vi "VL6180 GetRegister.vi"(7 "VL6180 Resource":T8 {"I2C Slave Address" format="%02x"}, 8 "error in":errorcluster, 10 "VL6180X Constants":T7 items=["IDENTIFICATION_MODEL_ID"=0, "IDENTIFICATION_MODEL_REV_MAJOR"=1, "IDENTIFICATION_MODEL_REV_MINOR"=2, "IDENTIFICATION_MODULE_REV_MAJOR"=3, "IDENTIFICATION_MODULE_REV_MINOR"=4, "IDENTIFICATION_DATE"=6, "IDENTIFICATION_TIME"=8, "SYSTEM_MODE_GPIO0"=16, "SYSTEM_MODE_GPIO1"=17, "SYSTEM_HISTORY_CTRL"=18, "SYSTEM_INTERRUPT_CONFIG_GPIO"=20, "SYSTEM_INTERRUPT_CLEAR"=21, "SYSTEM_FRESH_OUT_OF_RESET"=22, "SYSTEM_GROUPED_PARAMETER_HOLD"=23, "SYSRANGE_START"=24, "SYSRANGE_THRESH_HIGH"=25, "SYSRANGE_THRESH_LOW"=26, "SYSRANGE_INTERMEASUREMENT_PERIOD"=27, "SYSRANGE_MAX_CONVERGENCE_TIME"=28, "SYSRANGE_CROSSTALK_COMPENSATION_RATE"=30, "SYSRANGE_CROSSTALK_VALID_HEIGHT"=33, "SYSRANGE_EARLY_CONVERGENCE_ESTIMATE"=34, "SYSRANGE_PART_TO_PART_RANGE_OFFSET"=36, "SYSRANGE_RANGE_IGNORE_VALID_HEIGHT"=37, "SYSRANGE_RANGE_IGNORE_THRESHOLD"=38, "SYSRANGE_MAX_AMBIENT_LEVEL_MULT"=44, "SYSRANGE_RANGE_CHECK_ENABLES"=45, "SYSRANGE_VHV_RECALIBRATE"=46, "SYSRANGE_VHV_REPEAT_RATE"=49, "SYSALS_START"=56, "SYSALS_THRESH_HIGH"=58, "SYSALS_THRESH_LOW"=60, "SYSALS_INTERMEASUREMENT_PERIOD"=62, "SYSALS_ANALOGUE_GAIN"=63, "SYSALS_INTEGRATION_PERIOD"=64, "RESULT_RANGE_STATUS"=77, "RESULT_ALS_STATUS"=78, "RESULT_INTERRUPT_STATUS_GPIO"=79, "RESULT_ALS_VAL"=80, "RESULT_HISTORY_BUFFER"=82, "RESULT_RANGE_VAL"=98, "RESULT_RANGE_RAW"=100, "RESULT_RANGE_RETURN_RATE"=102, "RESULT_RANGE_REFERENCE_RATE"=104, "RESULT_RANGE_RETURN_SIGNAL_COUNT"=108, "RESULT_RANGE_REFERENCE_SIGNAL_COUNT"=112, "RESULT_RANGE_RETURN_AMB_COUNT"=116, "RESULT_RANGE_REFERENCE_AMB_COUNT"=120, "RESULT_RANGE_RETURN_CONV_TIME"=124, "RESULT_RANGE_REFERENCE_CONV_TIME"=128, "READOUT_AVERAGING_SAMPLE_PERIOD"=266, "FIRMWARE_BOOTUP"=281, "FIRMWARE_RESULT_SCALER"=288, "I2C_SLAVE_DEVICE_ADDRESS"=530, "INTERLEAVED_MODE_ENABLE"=675], 11 "LINX Resource":T1) -> (0 "error out":errorcluster, 2 "Data out":u8 format="%02x", 3 "LINX Resource":T1, 5 "VL6180 Resource":T8 {"I2C Slave Address" format="%02x"})   [LabVIEW 2014]
uses:
  VL6180 Resource.ctl
  VL6180X DEFS.ctl
  <vilib>/MakerHub/LINX/Private/Type Defs/LINX Ref.ctl
  <vilib>/MakerHub/LINX/Private/Type Defs/Platform.ctl
  <vilib>/MakerHub/LINX/Private/Type Defs/Interface.ctl
  <vilib>/MakerHub/LINX/Private/Device/Type Defs/LINX Device Config.ctl
  <vilib>/MakerHub/LINX/Private/Device/Type Defs/TCP Config.ctl
  <vilib>/MakerHub/LINX/Private/Device/Type Defs/Channels.ctl
  <vilib>/MakerHub/LINX/LMH-LINX.lvlib
  <vilib>/MakerHub/LINX/Private/Device/Device.lvlib
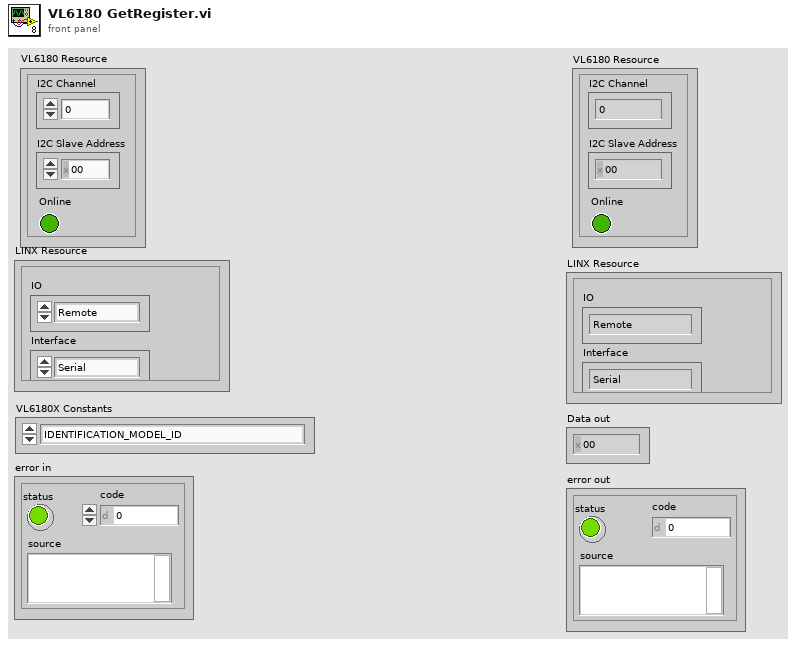
[diagram p1: front panel]
types:
  T1 = typedef "LMH-LINX.lvlib/LINX Ref.ctl" = cluster{"IO":T2, "Interface":T3, "LINX Device Config":T4}
  T2 = typedef "LMH-LINX.lvlib/Platform.ctl" = enum16{"Remote", "Local"}
  T3 = typedef "LMH-LINX.lvlib/Interface.ctl" = enum16{"Serial", "TCP"}
  T4 = typedef "LMH-LINX.lvlib/Device.lvlib/LINX Device Config.ctl" = cluster{"Interface":T3, "COM Port":refnum<visa-resource-name>, "TCP Configuration":T5, "Device Family":u8, "Device ID":u8, "Device Name":string, "TCP Ref":refnum<k5>, "Channels":T6}
  T5 = typedef "LMH-LINX.lvlib/Device.lvlib/TCP Config.ctl" = cluster{"IP Address":string, "Port":u16}
  T6 = typedef "LMH-LINX.lvlib/Channels.ctl" = cluster{"DI":u8[], "DO":u8[], "AI":u8[], "AO":u8[], "PWM":u8[], "QE":u8[], "UART":u8[], "I2C 2":u8[], "SPI":u8[], "CAN":u8[], "Servo":u8[], "AI Ref (V)":dbl, "AI Resolution (Bits)":u8, "AO Ref (V)":dbl, "AO Resolution (Bits)":u8}
  T7 = typedef "VL6180X DEFS.ctl" = u16
  T8 = typedef "VL6180 Resource.ctl" = cluster{"I2C Channel":u8, "I2C Slave Address":u8, "Online":bool}
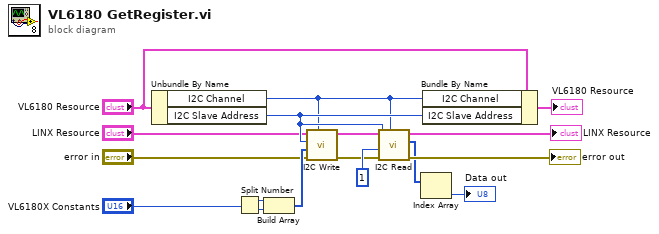
[diagram p0: block diagram]
diagram:
  n1 = Unbundle By Name("VL6180 Resource") -> ("I2C Channel"=w5:u8, "I2C Slave Address"=w6:u8)
  n2 = Split Number(x="VL6180X Constants") -> (hi(x)=w14:u8, lo(x)=w15:u8)
  n3 = Build Array(w14, w15) -> (w16:u8[])
  n4 = call <vilib>:"I2C Write.vi"("I2C Channel"=w5, "Error In"="error in", "Data"=w16, "I2C Slave Address (0)"=w6, "LINX Resource"="LINX Resource") -> ("Error Out"=w11:errorcluster, "LINX Resource"=w10:T1)  [unwired: 5 in]
  n5 = call <vilib>:"I2C Read.vi"("I2C Channel"=w5, "Error In"=w11, "Bytes To Read"=u8 1, "I2C Slave Address (0)"=w6, "LINX Resource"=w10) -> ("Error Out"=→"error out":errorcluster, "Data"=w13:u8[], "LINX Resource"=→"LINX Resource":T1)  [unwired: 4 in]
  n6 = Index Array(array=w13) -> (element=→"Data out":u8)  [unwired: 1 in]
  n7 = Bundle By Name(cluster="VL6180 Resource", "I2C Channel"=w5, "I2C Slave Address"=w6) -> (→"VL6180 Resource":T8)
